vi "Get Device ID.vi"(8 "Error In":errorcluster, 11 "LINX Resource":T1) -> (0 "Error Out":errorcluster, 2 "Device User ID":u16, 3 "LINX Resource":T1)   [LabVIEW 2011, in "LVH-LINX.lvlib"]
uses:
  LVH-LINX.lvlib
  Private/Type Defs/Error Type.ctl
  Private/Device/Device.lvlib
  Private/Type Defs/Platform.ctl
  Private/Type Defs/Interface.ctl
  Private/Device/Type Defs/TCP Config.ctl
  Private/Device/Type Defs/Channels.ctl
  Private/Device/Type Defs/LINX Device Config.ctl
  Private/Type Defs/LINX Ref.ctl
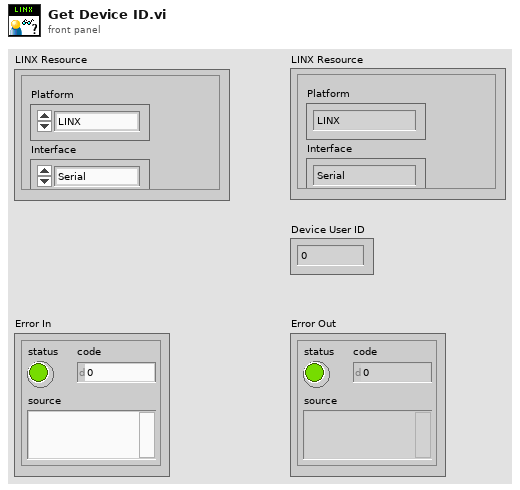
[diagram p1: front panel]
types:
  T1 = typedef "LVH-LINX.lvlib/LINX Ref.ctl" = cluster{"Platform":T2, "Interface":T3, "LINX Device Config":T4}
  T2 = typedef "LVH-LINX.lvlib/Platform.ctl" = enum16{"LINX", "myRIO"}
  T3 = typedef "LVH-LINX.lvlib/Interface.ctl" = enum16{"Serial", "TCP"}
  T4 = typedef "LVH-LINX.lvlib/Device.lvlib/LINX Device Config.ctl" = cluster{"Interface":T3, "COM Port":refnum<visa-resource-name>, "TCP Configuration":T5, "Device Family":u8, "Device ID":u8, "Device Name":string, "TCP Ref":refnum<k5>, "Channels":T6}
  T5 = typedef "LVH-LINX.lvlib/Device.lvlib/TCP Config.ctl" = cluster{"IP Address":string, "Port":u16}
  T6 = typedef "LVH-LINX.lvlib/Channels.ctl" = cluster{"DI Channels":u8[], "DO Channels":u8[], "AI":u8[], "AO":u8[], "PWM":u8[], "QE":u8[], "UART":u8[], "I2C 2":u8[], "SPI":u8[], "CAN":u8[], "AI Ref (V)":dbl, "AO Resolution (Bits)":u8, "AO Ref (V)":dbl}
  T7 = typedef "LVH-LINX.lvlib/Error Type.ctl" = enum16{"Unknown", "Timeout", "Corrupt Return Packet", "Unable To Connect", "Command Not Supported", "Channel DNE", "Invalid COM Config", "Firmware Version Mismatch", "myRIO Support"}
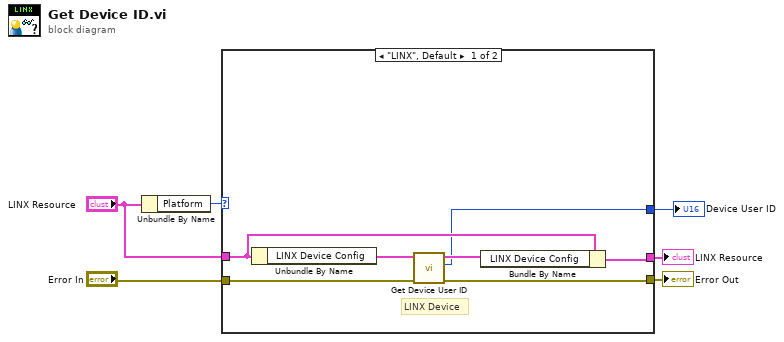
[diagram p0: block diagram]
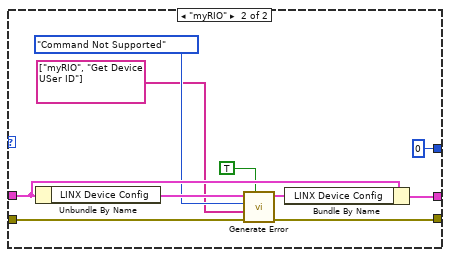
[diagram p2: hidden frame]
diagram:
  n1 = Unbundle By Name("LINX Resource") -> ("Platform"=w6:T2)
  n2 = case shown="\"LINX\", Default" w6 {
    tunnel: [w8 w19] -> w5
    tunnel: [w13 w18] -> w2
    tunnel: "Error In" -> [w9 w20]
    tunnel: "LINX Resource" -> [w12 w23]
    tunnel: [w7 u16 0 ("Device User ID")] -> w1
    frame "LINX", Default {
      # "LINX Device"
      n3 = Unbundle By Name(w12) -> ("LINX Device Config"=w10:T4)
      n4 = call "Get Device User ID.vi"("Error In"=w9, "LINX Device Config"=w10) -> ("Error Out"=w8:errorcluster, "Device User ID"=w7:u16, "LINX Device Config"=w11:T4)  [unwired: 7 in]
      n5 = Bundle By Name(cluster=w12, "LINX Device Config"=w11) -> (w13:T1)
    }
    frame "myRIO" {
      n6 = Unbundle By Name(w23) -> ("LINX Device Config"=w22:T4)
      n7 = call "Generate Error.vi"("Is Warning? (False)"=TRUE, "Error In"=w20, "Arguments"=string[] ["myRIO", "Get Device USer ID"], "Error Type"=Error_Type."Command Not Supported", "LINX Device Config"=w22) -> ("Error Out"=w19:errorcluster, "LINX Device Config"=w21:T4)  [unwired: 5 in]
      n8 = Bundle By Name(cluster=w23, "LINX Device Config"=w21) -> (w18:T1)
    }
  }
  "Error Out" <- w5
  "LINX Resource" <- w2
  "Device User ID" <- w1
